vi "mkSendSerialCmd.vi"(8 "error in (no error)":errorcluster, 10 "String":string, 11 "IMAQ Refnum in":refnum<k11>) -> (0 "error out":errorcluster, 1 "total error count":i16, 2 "String Read":string, 3 "IMAQ Refnum out":refnum<k11>)   [LabVIEW 2011]
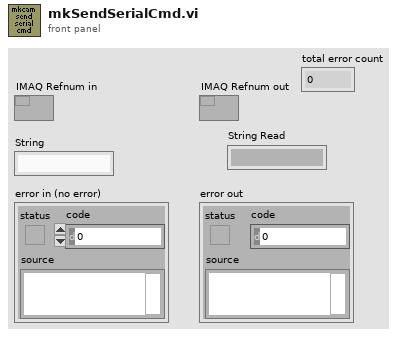
[diagram p1: front panel]
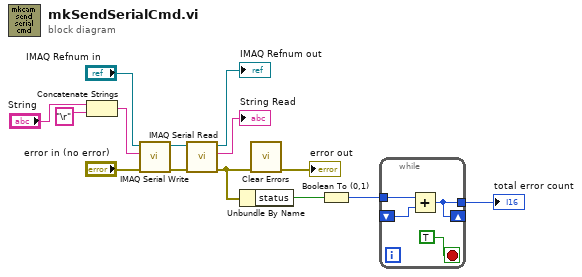
[diagram p0: block diagram]
diagram:
  n1 = Concatenate Strings("String", "\r" ("string")) -> (w6:string)
  n2 = call <vilib>:"IMAQ Serial Write.vi"("error in (no error)"="error in (no error)", "String to write"=w6, "IMAQ Session In"="IMAQ Refnum in") -> ("error out"=w12:errorcluster, "IMAQ Session Out"=w13:refnum<k11>)  [unwired: 5 in]
  n3 = call <vilib>:"IMAQ Serial Read.vi"("error in (no error)"=w12, "IMAQ Session In"=w13) -> ("error out"=w4:errorcluster, "String Read"=→"String Read":string, "IMAQ Session Out"=→"IMAQ Refnum out":refnum<k11>)  [unwired: 4 in, 1 out]
  n4 = Unbundle By Name(w4) -> ("status"=w3:bool)
  n5 = call <vilib>:"Clear Errors.vi"("error in (no error)"=w4) -> ("error out"=→"error out":errorcluster)  [unwired: 6 in]
  n6 = Boolean To (0,1)(Boolean=w3) -> (0, 1=w2:i16)
  n7 = while {
    tunnel: w2 -> [w17]
    shift-right: [w15] -> _
    shift-left: _ -> [w16]
    tunnel: [w15] -> w1
    stop <- TRUE stop-if-true
    n8 = Add(x=w17, y=w16) -> (x+y=w15:i16)
  }
  "total error count" <- w1
